vi "Close.vi"(8 "error in (no error)":errorcluster caption="错误输入（无错误）", 11 "Serial 输入":refnum<class "Serial.lvclass"> caption="DNL_LabVIEW Object in") -> (0 "error out":errorcluster caption="错误输出", 3 "Serial 输出":refnum<class "Serial.lvclass"> caption="DNL_LabVIEW Object out")   [LabVIEW 2012, in "Serial.lvclass"]
uses:
  Serial.lvclass
  PComm/PCOMM.lvlib
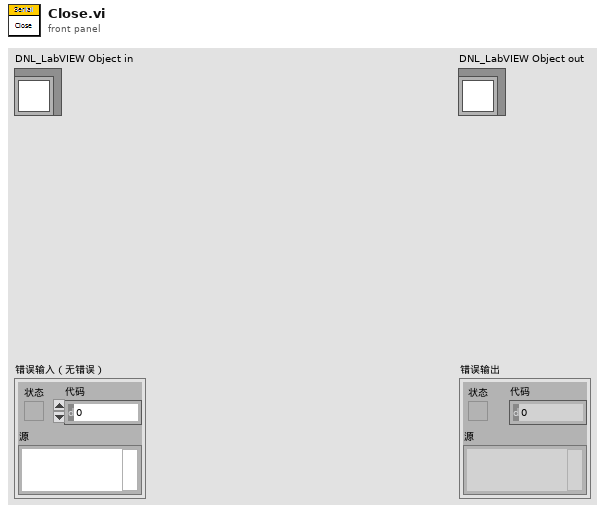
[diagram p1: front panel]
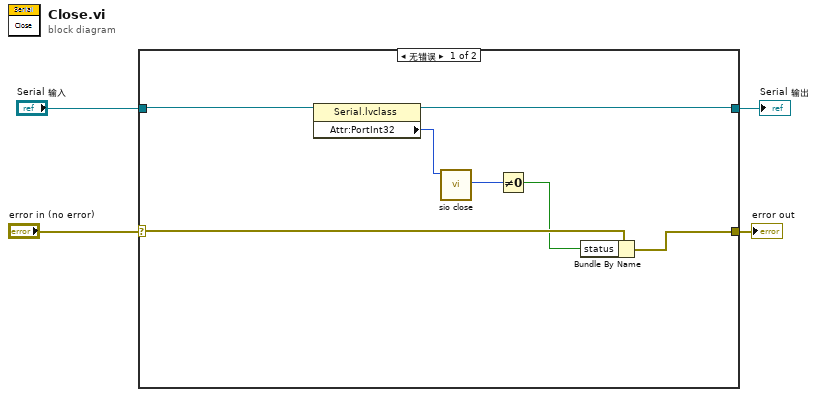
[diagram p0: block diagram]
diagram:
  n1 = case shown="无错误" "error in (no error)" {
    selector: "error in (no error)" -> [w7 w13]
    tunnel: [w5 w13] -> w3
    tunnel: [w9 w12] -> w1
    tunnel: "Serial 输入" -> [w11 w12]
    frame No Error {
      n2 = property class="Serial.lvclass"(reference=w11) -> (reference out=w9:refnum<class "Serial.lvclass">, "Attr:PortInt32"=w10:i32)  [unwired: 1 in, 1 out]
      n3 = call "sio close.vi"("port"=w10) -> ("function return"=w8:i32)  [unwired: 8 in, 1 out]
      n4 = Not Equal To 0?(x=w8) -> (x != 0?=w6:bool)
      n5 = Bundle By Name(cluster=w7, "status"=w6) -> (w5:errorcluster)
    }
    frame Error {
    }
  }
  "error out" <- w3
  "Serial 输出" <- w1
